vi "Update Array.vi"(8 "error in (no error)":errorcluster, 10 "Array":dbl[](array[numeric]), 11 "Example View In":refnum<class "Example GUI View Actor.lvclass">) -> (0 "error out":errorcluster, 3 "Example View Out":refnum<class "Example GUI View Actor.lvclass">)   [LabVIEW 2017, in "Example GUI View Actor.lvlib" / "Example GUI View Actor.lvclass"]
uses:
  Example GUI View Actor.lvclass
  Example GUI View Actor.lvclass/Example GUI View Actor.ctl
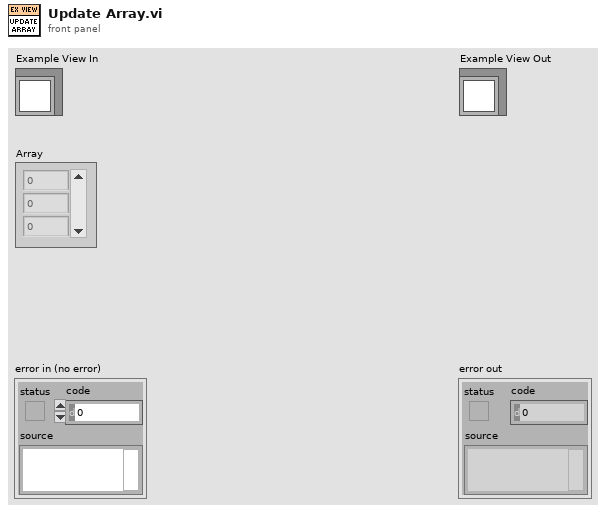
[diagram p1: front panel]
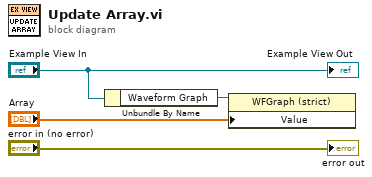
[diagram p0: block diagram]
diagram:
  n1 = Unbundle By Name("Example View In") -> ("Waveform Graph"=w2:refnum<vi>)
  n2 = property class="WFGraph (strict)"(reference=w2, "Value"="Array") -> ()  [unwired: 1 in, 2 out]
  "error out" <- "error in (no error)"
  "Example View Out" <- "Example View In"
